vi "Init.vi"(8 "error in (no error)":errorcluster, 11 "Data in":refnum<class "Var Bus.lvclass">) -> (0 "error out":errorcluster, 3 "Data out":refnum<class "Var Bus.lvclass">)   [LabVIEW 2021, in "Var Bus.lvclass"]
uses:
  Var Bus.lvclass
  Var Index/Var_Index.lvclass
  <vilib>/Utility/error.llb/DialogType.ctl
  Var Access/Var_Access.lvclass
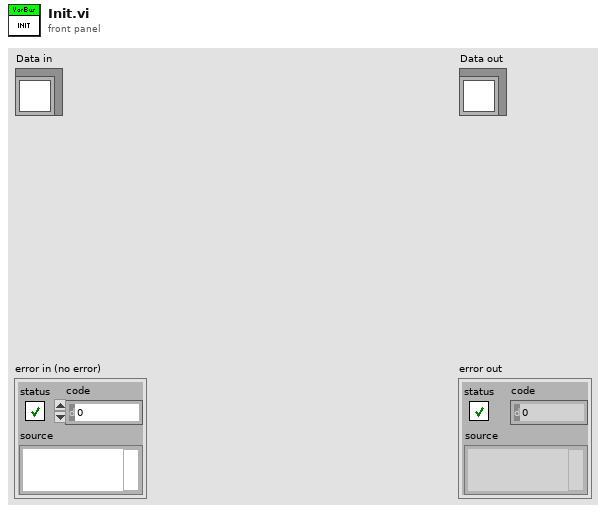
[diagram p1: front panel]
types:
  T1 = typedef "DialogType.ctl" = u16
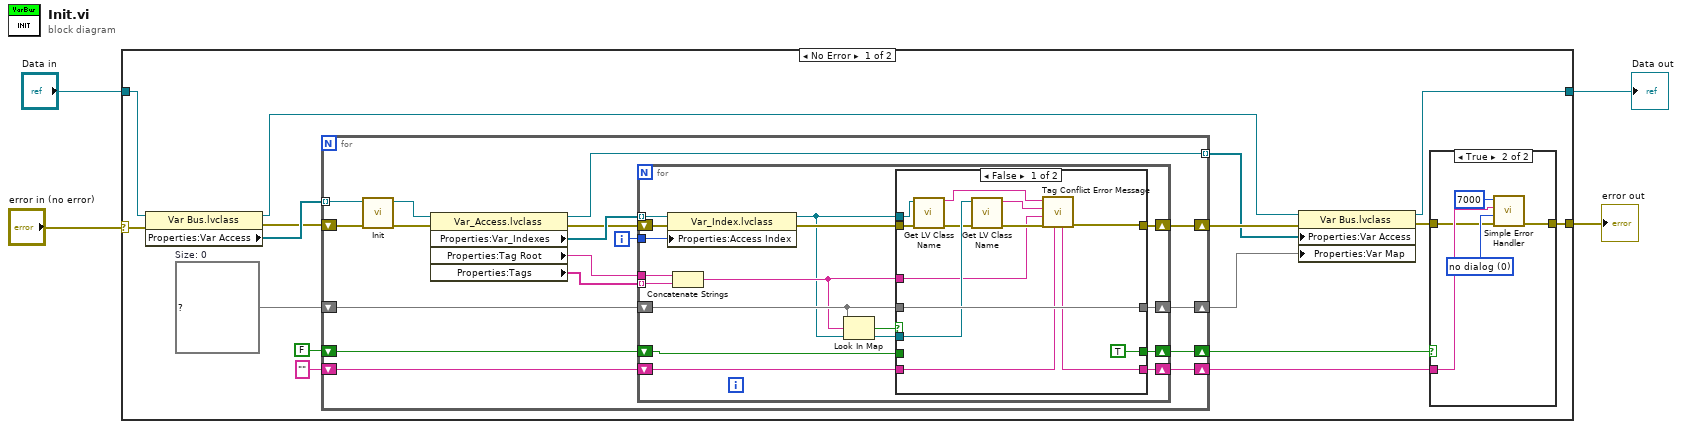
[diagram p0: block diagram]
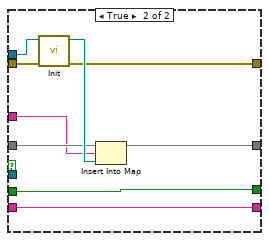
[diagram p3: hidden frame]
diagram:
  n1 = case shown="No Error" "error in (no error)" {
    selector: "error in (no error)" -> [w20 w83]
    tunnel: "Data in" -> [w19 w84]
    tunnel: [w6 w83] -> w2
    tunnel: [w13 w84] -> w1
    frame No Error {
      w12 = map{string, refnum<class "Var_Index.lvclass">} {}  # Size: 0
      n2 = property class="Var Bus.lvclass"(reference=w19, error in=w20) -> (reference out=w14:refnum<class "Var Bus.lvclass">, error out=w17:errorcluster, "Properties:Var Access"=w18:refnum<class "Var_Access.lvclass">[])
      n3 = for {
        tunnel: w18 -> [w42] mode=indexing
        shift-right: [w31] -> w16
        shift-left: w17 -> [w43]
        tunnel: [w39] -> w15 mode=indexing
        shift-right: [w36] -> w11
        shift-left: w12 -> [w35]
        shift-right: [w30] -> w5
        shift-left: "" -> [w29]
        shift-right: [w28] -> w8
        shift-left: FALSE -> [w27]
        i -> [w32]
        n4 = call-dynamic "Init.vi"("error in (no error)"=w43, "Data in"=w42) -> ("error out"=w41:errorcluster, "Data out"=w40:refnum<class "Var_Access.lvclass">)  [unwired: 8 in]
        n5 = property class="Var_Access.lvclass"(reference=w40, error in=w41) -> (reference out=w39:refnum<class "Var_Access.lvclass">, error out=w33:errorcluster, "Properties:Var_Indexes"=w34:refnum<class "Var_Index.lvclass">[], "Properties:Tag Root"=w38:string, "Properties:Tags"=w37:string[])
        n6 = for {
          tunnel: w38 -> [w60]
          tunnel: w37 -> [w59] mode=indexing
          tunnel: w34 -> [w57] mode=indexing
          shift-right: [w58] -> w36
          shift-left: w35 -> [w53]
          tunnel: w32 -> [w55]
          shift-right: [w50] -> w31
          shift-left: w33 -> [w56]
          shift-right: [w47] -> w30
          shift-left: w29 -> [w46]
          shift-right: [w45] -> w28
          shift-left: w27 -> [w44]
          n7 = property class="Var_Index.lvclass"(reference=w57, error in=w56, "Properties:Access Index"=w55) -> (reference out=w51:refnum<class "Var_Index.lvclass">, error out=w54:errorcluster)
          n8 = Concatenate Strings(w60, w59) -> (w52:string)
          n9 = Look In Map(map=w53, key=w52, default value=w51) -> (key not found?=w49:bool, value=w48:refnum<class "Var_Index.lvclass">)
          n10 = case shown="False" w49 {
            tunnel: [w73 w82] -> w58
            tunnel: w54 -> [w71 w81]
            tunnel: w53 -> [w73 w79]
            tunnel: w52 -> [w64 w78]
            tunnel: w51 -> [w70 w77]
            tunnel: [w67 w76] -> w50
            tunnel: w48 -> [w72 _]
            tunnel: [w63 w75] -> w47
            tunnel: w46 -> [w62 w75]
            tunnel: [TRUE w74] -> w45
            tunnel: w44 -> [_ w74]
            frame False {
              n11 = call <vilib>:"Get LV Class Name.vi"("error in (no error)"=w71, "object"=w70) -> ("error out"=w69:errorcluster, "class name"=w66:string)  [unwired: 8 in]
              n12 = call <vilib>:"Get LV Class Name.vi"("error in (no error)"=w69, "object"=w72) -> ("error out"=w68:errorcluster, "class name"=w65:string)  [unwired: 8 in]
              n13 = call "Tag Conflict Error Message.vi"("Previous Error Message"=w62, "error in (no error)"=w68, "Tag Name"=w64, "Conflict Class"=w65, "Original Class"=w66) -> ("error out"=w67:errorcluster, "Error Message"=w63:string)  [unwired: 5 in]
            }
            frame True {
              n14 = call-dynamic "Init.vi"("error in (no error)"=w81, "Data in"=w77) -> ("error out"=w76:errorcluster, "Data out"=w80:refnum<class "Var_Index.lvclass">)  [unwired: 8 in]
              n15 = Insert Into Map(map in=w79, key=w78, value=w80) -> (map out=w82:map{string, refnum<class "Var_Index.lvclass">})  [unwired: 2 out]
            }
          }
        }
      }
      n16 = property class="Var Bus.lvclass"(reference=w14, error in=w16, "Properties:Var Access"=w15, "Properties:Var Map"=w11) -> (reference out=w13:refnum<class "Var Bus.lvclass">, error out=w7:errorcluster)
      n17 = case shown="True" w8 {
        tunnel: w7 -> [w21 w22]
        tunnel: [w21 w26] -> w6
        tunnel: w5 -> [_ w23]
        frame False {
        }
        frame True {
          w25 = T1 0 items=["no dialog", "OK message", "continue or stop message", "OK message + warnings", "continue/stop + warnings"] ("type of dialog (OK msg:1)")
          n18 = call <vilib>:"Simple Error Handler.vi"("error code (no error:0)"=7000, "error source (\" \")"=w23, "type of dialog (OK msg:1)"=w25, "error in (no error)"=w22) -> ("error out"=w26:errorcluster)  [unwired: 1 in, 4 out]
        }
      }
    }
    frame Error {
    }
  }
  "error out" <- w2
  "Data out" <- w1
